vi "UiSchematic_gas.vi"() -> ()   [LabVIEW 2011]
uses:
  Pumpe.ctl
  Output - Cluster gas.ctl
panel:
  out "B2G1 HR V1":bool
  out "Fab2 MR V1":bool
  out "B2G1 MR V1":bool
  out "B2G2 T2 V1":bool
  out "B2G2 MR V1":bool
  out "B2G1 T2 V1":bool
  out "Fab1 BL V1":bool
  out "Fab1 HR V1":bool
  out "Fab1 MR V1":bool
  out "Fab2 HR V1":bool
  out "DS-2 [bar]":dbl format="%.4g"
  out "GZ-1 [l]":dbl format="%.2f"
  out "DS-1 [bar]":dbl format="%.4g"
  out "TS-1 [°C]":dbl format="%.2g"
  out "cRio":timestamp
  out "GM P-2":bool
  out "PC":timestamp
  in  "stop cRIO":bool
  out "GM V-1":bool
  out "GM V-4":bool
  out "GM V-3":bool
  out "GM V-2":bool
  out "GA1":timestamp caption="GA-1"
  out "h2 [%]":dbl format="%.2g"
  out "co2 [%]":dbl format="%.2g"
  out "ch4 [%]":dbl format="%.2g"
  out "GM P-1":T1
  out "B2G1 HR V1.1":bool
  out "Fab2 MR V1.1":bool
  out "B2G1 MR V1.1":bool
  out "B2G2 T2 V1.1":bool
  out "B2G2 MR V1.1":bool
  out "B2G1 T2 V1.1":bool
  out "Fab1 BL V1.1":bool
  out "Fab1 HR V1.1":bool
  out "Fab1 MR V1.1":bool
  out "Fab2 HR V1.1":bool
  in  "Output Var gas":refnum<k21>="ni.var.psp://10.27.40.21/variables - gas/data - network - gas"
  in  "stop":bool
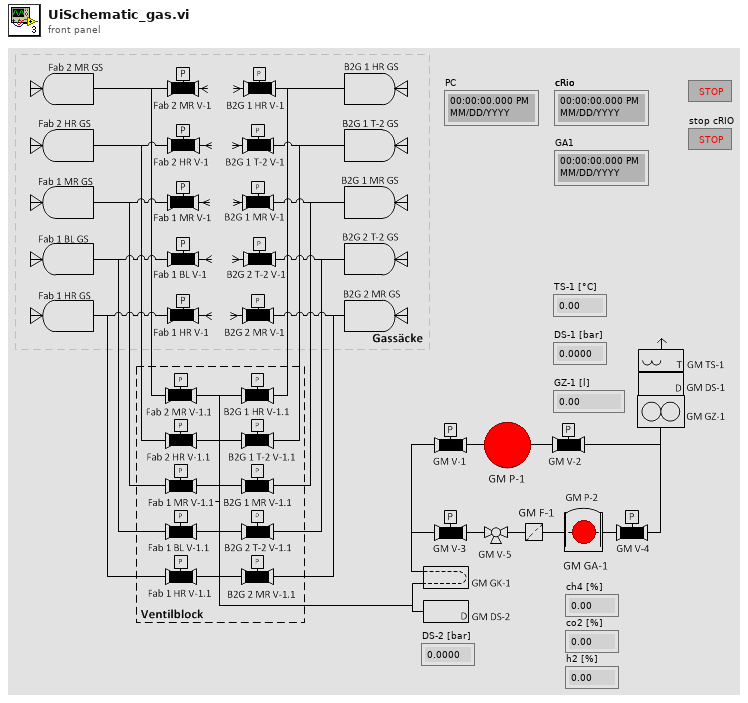
[diagram p1: front panel]
types:
  T1 = typedef "Pumpe.ctl" = bool
  T2 = typedef "Output - Cluster gas.ctl" = cluster{"B2G2 MR V1.1 AUF":bool, "B2G2 MR V1.1 ZU":bool, "B2G2 MR V1 AUF":bool, "B2G2 MR V1 ZU":bool, "B2G1 T2 V1 AUF":bool, "B2G1 T2 V1 ZU":bool, "B2G1 T2 V1.1 AUF":bool, "B2G1 T2 V1.1 ZU":bool, "B2G2 T2 V1 AUF":bool, "B2G2 T2 V1 ZU":bool, "B2G2 T2 V1.1 ZU":bool, "B2G2 T2 V1.1 AUF":bool, "B2G1 MR V1 AUF":bool, "B2G1 MR V1 ZU":bool, "B2G1 MR V1.1 AUF":bool, "B2G1 MR V1.1 ZU":bool, "B2G1 HR V1 AUF":bool, "B2G1 HR V1 ZU":bool, "B2G1 HR V1.1 AUF":bool, "B2G1 HR V1.1 ZU":bool, "Fab1 HR V1 AUF":bool, "Fab1 HR V1 ZU":bool, "Fab1 HR V1.1 AUF":bool, "Fab1 HR V1.1 ZU":bool, "Fab1 MR V1 AUF":bool, "Fab1 MR V1 ZU":bool, "Fab1 MR V1.1 AUF":bool, "Fab1 MR V1.1 ZU":bool, "Fab1 BL V1 AUF":bool, "Fab1 BL V1 ZU":bool, "Fab1 BL V1.1 AUF":bool, "Fab1 BL V1.1 ZU":bool, "Fab2 HR V1 AUF":bool, "Fab2 HR V1 ZU":bool, "Fab2 HR V1.1 AUF":bool, "Fab2 HR V1.1 ZU":bool, "Fab2 MR V1 AUF":bool, "Fab2 MR V1 ZU":bool, "Fab2 MR V1.1 AUF":bool, "Fab2 MR V1.1 ZU":bool, "GA1 ch4":dbl, "GA1 co2":dbl, "GA1 h2":dbl, "GM P1 RUN":bool, "GA1 timestamp":timestamp, "GM V-1 AUF":bool, "GM V-1 ZU":bool, "GM V-2 AUF":bool, "GM V-2 ZU":bool, "GM V-3 AUF":bool, "GM V-3 ZU":bool, "GM V-4 AUF":bool, "GM V-4 ZU":bool, "GM P2 RUN":bool, "GM GZ-1 [l]":dbl, "GM DS-2 [bar]":dbl, "GM DS-1 [bar]":dbl, "GM TS-1 [°C]":dbl}
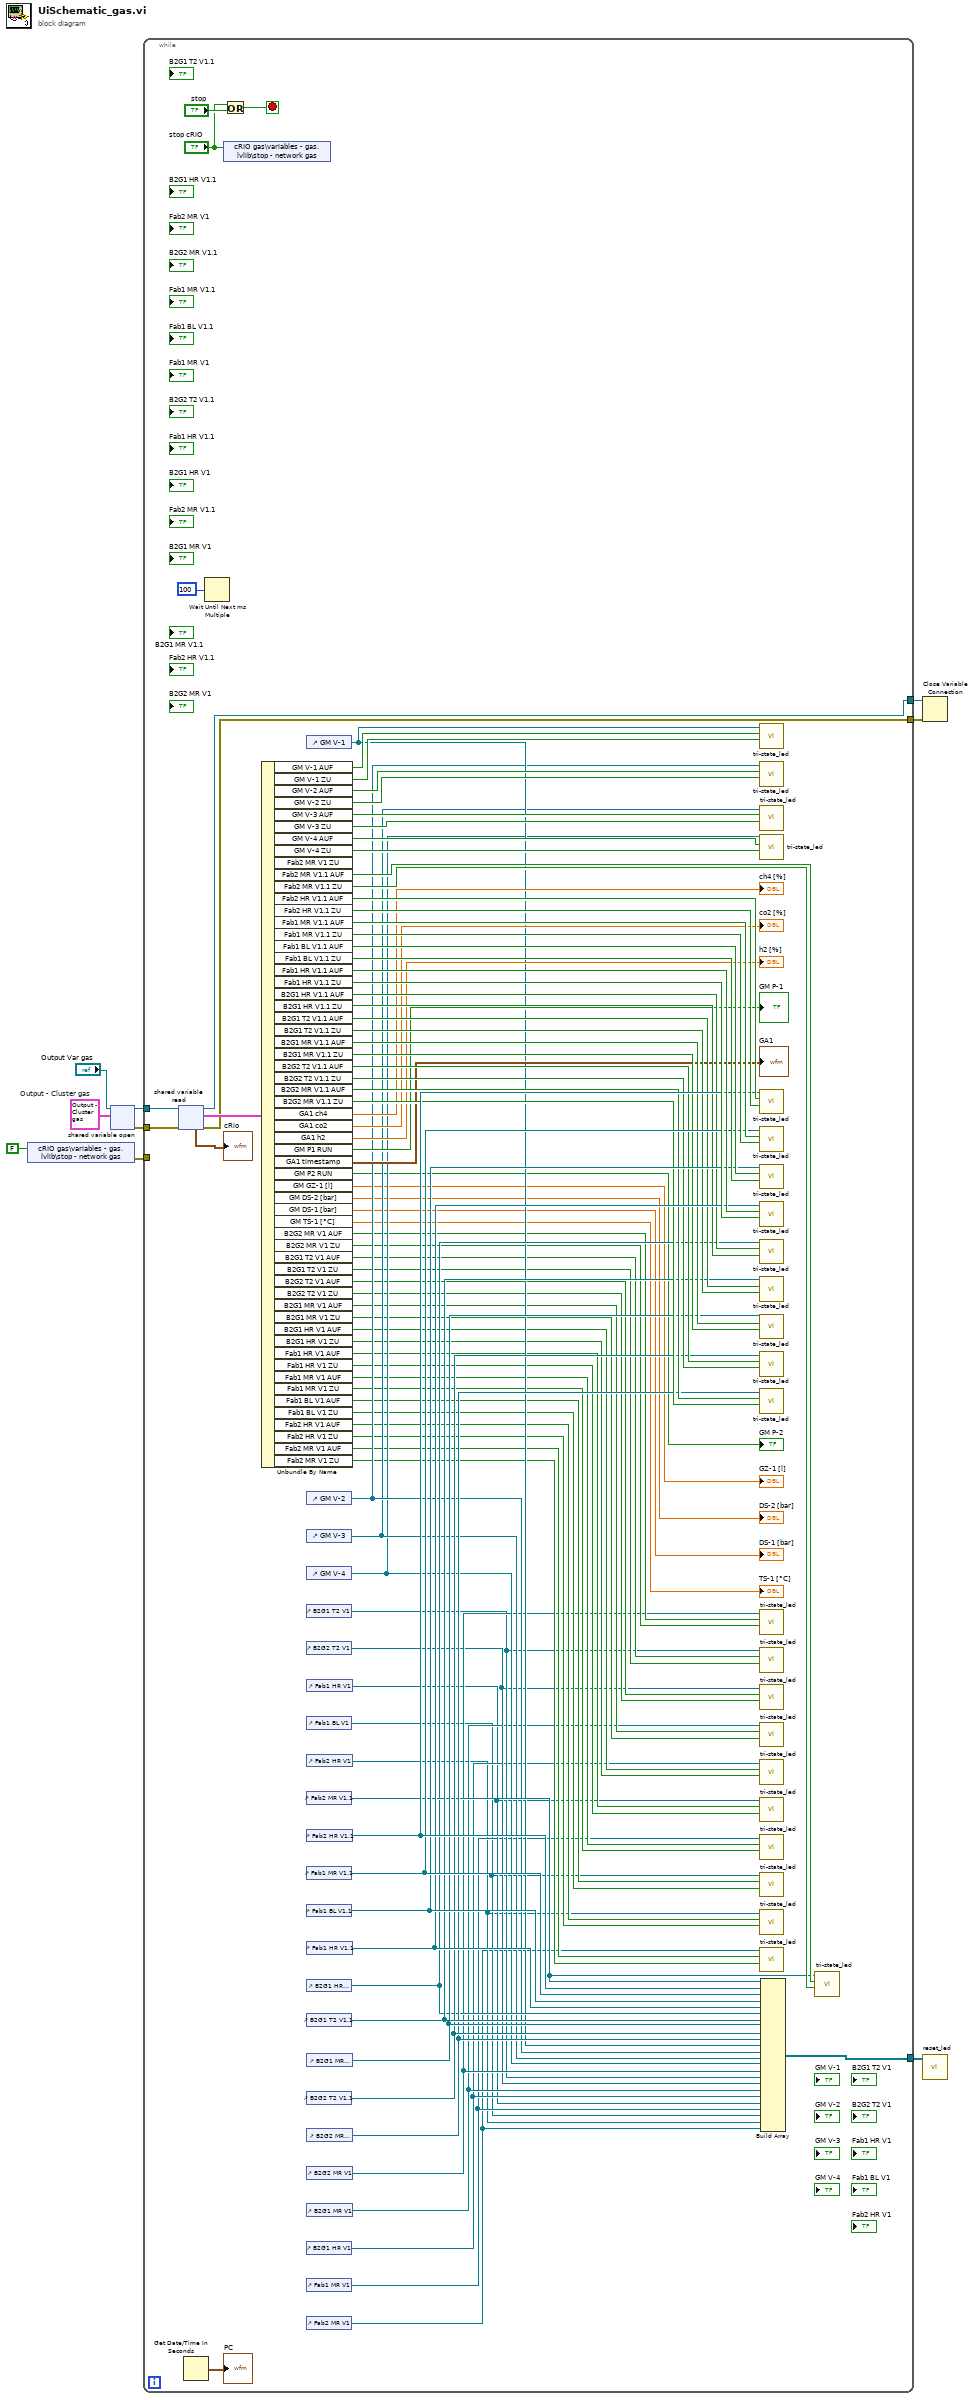
[diagram p0: block diagram]
diagram:
  w6 = T2 {"B2G2 MR V1.1 AUF"=FALSE, "B2G2 MR V1.1 ZU"=FALSE, "B2G2 MR V1 AUF"=FALSE, "B2G2 MR V1 ZU"=FALSE, "B2G1 T2 V1 AUF"=FALSE, "B2G1 T2 V1 ZU"=FALSE, "B2G1 T2 V1.1 AUF"=FALSE, "B2G1 T2 V1.1 ZU"=FALSE, "B2G2 T2 V1 AUF"=FALSE, "B2G2 T2 V1 ZU"=FALSE, "B2G2 T2 V1.1 ZU"=FALSE, "B2G2 T2 V1.1 AUF"=FALSE, "B2G1 MR V1 AUF"=FALSE, "B2G1 MR V1 ZU"=FALSE, "B2G1 MR V1.1 AUF"=FALSE, "B2G1 MR V1.1 ZU"=FALSE, "B2G1 HR V1 AUF"=FALSE, "B2G1 HR V1 ZU"=FALSE, "B2G1 HR V1.1 AUF"=FALSE, "B2G1 HR V1.1 ZU"=FALSE, "Fab1 HR V1 AUF"=FALSE, "Fab1 HR V1 ZU"=FALSE, "Fab1 HR V1.1 AUF"=FALSE, "Fab1 HR V1.1 ZU"=FALSE, "Fab1 MR V1 AUF"=FALSE, "Fab1 MR V1 ZU"=FALSE, "Fab1 MR V1.1 AUF"=FALSE, "Fab1 MR V1.1 ZU"=FALSE, "Fab1 BL V1 AUF"=FALSE, "Fab1 BL V1 ZU"=FALSE, "Fab1 BL V1.1 AUF"=FALSE, "Fab1 BL V1.1 ZU"=FALSE, "Fab2 HR V1 AUF"=FALSE, "Fab2 HR V1 ZU"=FALSE, "Fab2 HR V1.1 AUF"=FALSE, "Fab2 HR V1.1 ZU"=FALSE, "Fab2 MR V1 AUF"=FALSE, "Fab2 MR V1 ZU"=FALSE, "Fab2 MR V1.1 AUF"=FALSE, "Fab2 MR V1.1 ZU"=FALSE, "GA1 ch4"=0.0, "GA1 co2"=0.0, "GA1 h2"=0.0, "GM P1 RUN"=FALSE, "GA1 timestamp"=timestamp(0 s since 1904-01-01), "GM V-1 AUF"=FALSE, "GM V-1 ZU"=FALSE, "GM V-2 AUF"=FALSE, "GM V-2 ZU"=FALSE, "GM V-3 AUF"=FALSE, "GM V-3 ZU"=FALSE, "GM V-4 AUF"=FALSE, "GM V-4 ZU"=FALSE, "GM P2 RUN"=FALSE, "GM GZ-1 [l]"=0.0, "GM DS-2 [bar]"=0.0, "GM DS-1 [bar]"=0.0, "GM TS-1 [°C]"=0.0}  # Output - Cluster gas
  n1 = shared-variable "cRIO gas\\variables - gas.lvlib\\stop - network gas"(FALSE ("stop - network gas")) -> (error out=w2:errorcluster)  [unwired: 1 in]
  n2 = shared-variable-open("Output Var gas", w6) -> (w4:refnum<k21>, w3:errorcluster)  [unwired: 2 in]
  n3 = while {
    tunnel: w4 -> [w103]
    tunnel: [w102] -> w8
    tunnel: w3 -> [w100]
    tunnel: [w99] -> w7
    tunnel: [w83] -> w5
    tunnel: w2 -> [_]
    stop <- w49 stop-if-true
    n4 = shared-variable-read(w103, w100) -> (w102:refnum<k21>, w99:errorcluster, w101:T2, →"cRio":timestamp)
    n5 = Get Date/Time In Seconds() -> (seconds since 1Jan1904=→"PC":timestamp)
    n6 = Wait Until Next ms Multiple(millisecond multiple=u32 100) -> ()  [unwired: 1 out]
    n7 = Or(x="stop cRIO", y="stop") -> (x .or. y?=w49:bool)
    n8 = shared-variable "cRIO gas\\variables - gas.lvlib\\stop - network gas"("stop cRIO") -> ()  [unwired: 1 in, 1 out]
    n9 = Unbundle By Name(w101) -> ("GM V-1 AUF"=w61:bool, "GM V-1 ZU"=w60:bool, "GM V-2 AUF"=w59:bool, "GM V-2 ZU"=w58:bool, "GM V-3 AUF"=w57:bool, "GM V-3 ZU"=w56:bool, "GM V-4 AUF"=w55:bool, "GM V-4 ZU"=w54:bool, "Fab2 MR V1.1 AUF"=w97:bool, "Fab2 MR V1.1 ZU"=w96:bool, "Fab2 HR V1.1 AUF"=w95:bool, "Fab2 HR V1.1 ZU"=w94:bool, "Fab1 MR V1.1 AUF"=w93:bool, "Fab1 MR V1.1 ZU"=w92:bool, "Fab1 BL V1.1 AUF"=w91:bool, "Fab1 BL V1.1 ZU"=w90:bool, "Fab1 HR V1.1 AUF"=w89:bool, "Fab1 HR V1.1 ZU"=w88:bool, "B2G1 HR V1.1 AUF"=w82:bool, "B2G1 HR V1.1 ZU"=w81:bool, "B2G1 T2 V1.1 AUF"=w80:bool, "B2G1 T2 V1.1 ZU"=w79:bool, "B2G1 MR V1.1 AUF"=w78:bool, "B2G1 MR V1.1 ZU"=w77:bool, "B2G2 T2 V1.1 AUF"=w76:bool, "B2G2 T2 V1.1 ZU"=w75:bool, "B2G2 MR V1.1 AUF"=w74:bool, "B2G2 MR V1.1 ZU"=w73:bool, "GA1 ch4"=→"ch4 [%]":dbl, "GA1 co2"=→"co2 [%]":dbl, "GA1 h2"=→"h2 [%]":dbl, "GM P1 RUN"=→"GM P-1":bool, "GA1 timestamp"=→"GA1":timestamp, "GM P2 RUN"=→"GM P-2":bool, "GM GZ-1 [l]"=→"GZ-1 [l]":dbl, "GM DS-2 [bar]"=→"DS-2 [bar]":dbl, "GM DS-1 [bar]"=→"DS-1 [bar]":dbl, "GM TS-1 [°C]"=→"TS-1 [°C]":dbl, "B2G2 MR V1 AUF"=w39:bool, "B2G2 MR V1 ZU"=w38:bool, "B2G1 T2 V1 AUF"=w37:bool, "B2G1 T2 V1 ZU"=w36:bool, "B2G2 T2 V1 AUF"=w35:bool, "B2G2 T2 V1 ZU"=w34:bool, "B2G1 MR V1 AUF"=w33:bool, "B2G1 MR V1 ZU"=w32:bool, "B2G1 HR V1 AUF"=w31:bool, "B2G1 HR V1 ZU"=w30:bool, "Fab1 HR V1 AUF"=w29:bool, "Fab1 HR V1 ZU"=w28:bool, "Fab1 MR V1 AUF"=w27:bool, "Fab1 MR V1 ZU"=w26:bool, "Fab1 BL V1 AUF"=w25:bool, "Fab1 BL V1 ZU"=w24:bool, "Fab2 HR V1 AUF"=w23:bool, "Fab2 HR V1 ZU"=w22:bool, "Fab2 MR V1 AUF"=w21:bool, "Fab2 MR V1 ZU"=w20:bool)  [unwired: 1 out]
    n10 = control-ref of="GM V-1"() -> (w53:refnum<vi>)
    n11 = control-ref of="GM V-2"() -> (w52:refnum<vi>)
    n12 = control-ref of="GM V-3"() -> (w51:refnum<vi>)
    n13 = control-ref of="GM V-4"() -> (w50:refnum<vi>)
    n14 = control-ref of="B2G1 T2 V1"() -> (w18:refnum<vi>)
    n15 = control-ref of="B2G2 T2 V1"() -> (w17:refnum<vi>)
    n16 = control-ref of="Fab1 BL V1"() -> (w12:refnum<vi>)
    n17 = control-ref of="Fab2 MR V1.1"() -> (w68:refnum<vi>)
    n18 = control-ref of="Fab1 MR V1.1"() -> (w86:refnum<vi>)
    n19 = control-ref of="Fab1 BL V1.1"() -> (w85:refnum<vi>)
    n20 = control-ref of="B2G1 HR V1.1"() -> (w67:refnum<vi>)
    n21 = control-ref of="B2G1 T2 V1.1"() -> (w72:refnum<vi>)
    n22 = control-ref of="B2G2 T2 V1.1"() -> (w70:refnum<vi>)
    n23 = control-ref of="B2G1 HR V1"() -> (w15:refnum<vi>)
    n24 = control-ref of="Fab1 MR V1"() -> (w13:refnum<vi>)
    n25 = control-ref of="Fab2 MR V1"() -> (w10:refnum<vi>)
    n26 = control-ref of="Fab1 HR V1"() -> (w14:refnum<vi>)
    n27 = control-ref of="Fab2 HR V1"() -> (w11:refnum<vi>)
    n28 = control-ref of="Fab2 HR V1.1"() -> (w87:refnum<vi>)
    n29 = control-ref of="Fab1 HR V1.1"() -> (w84:refnum<vi>)
    n30 = control-ref of="B2G1 MR V1.1"() -> (w71:refnum<vi>)
    n31 = control-ref of="B2G2 MR V1.1"() -> (w69:refnum<vi>)
    n32 = control-ref of="B2G2 MR V1"() -> (w19:refnum<vi>)
    n33 = control-ref of="B2G1 MR V1"() -> (w16:refnum<vi>)
    n34 = call "tri-state_led.vi"("CLOSE"=w60, "OPEN"=w61, "ref in"=w53) -> ()  [unwired: 9 in]
    n35 = call "tri-state_led.vi"("CLOSE"=w58, "OPEN"=w59, "ref in"=w52) -> ()  [unwired: 9 in]
    n36 = call "tri-state_led.vi"("CLOSE"=w56, "OPEN"=w57, "ref in"=w51) -> ()  [unwired: 9 in]
    n37 = call "tri-state_led.vi"("CLOSE"=w54, "OPEN"=w55, "ref in"=w50) -> ()  [unwired: 9 in]
    n38 = call "tri-state_led.vi"("CLOSE"=w94, "OPEN"=w95, "ref in"=w87) -> ()  [unwired: 9 in]
    n39 = call "tri-state_led.vi"("CLOSE"=w92, "OPEN"=w93, "ref in"=w86) -> ()  [unwired: 9 in]
    n40 = call "tri-state_led.vi"("CLOSE"=w90, "OPEN"=w91, "ref in"=w85) -> ()  [unwired: 9 in]
    n41 = call "tri-state_led.vi"("CLOSE"=w88, "OPEN"=w89, "ref in"=w84) -> ()  [unwired: 9 in]
    n42 = call "tri-state_led.vi"("CLOSE"=w81, "OPEN"=w82, "ref in"=w67) -> ()  [unwired: 9 in]
    n43 = call "tri-state_led.vi"("CLOSE"=w79, "OPEN"=w80, "ref in"=w72) -> ()  [unwired: 9 in]
    n44 = call "tri-state_led.vi"("CLOSE"=w77, "OPEN"=w78, "ref in"=w71) -> ()  [unwired: 9 in]
    n45 = call "tri-state_led.vi"("CLOSE"=w75, "OPEN"=w76, "ref in"=w70) -> ()  [unwired: 9 in]
    n46 = call "tri-state_led.vi"("CLOSE"=w73, "OPEN"=w74, "ref in"=w69) -> ()  [unwired: 9 in]
    n47 = call "tri-state_led.vi"("CLOSE"=w38, "OPEN"=w39, "ref in"=w19) -> ()  [unwired: 9 in]
    n48 = call "tri-state_led.vi"("CLOSE"=w36, "OPEN"=w37, "ref in"=w18) -> ()  [unwired: 9 in]
    n49 = call "tri-state_led.vi"("CLOSE"=w34, "OPEN"=w35, "ref in"=w17) -> ()  [unwired: 9 in]
    n50 = call "tri-state_led.vi"("CLOSE"=w32, "OPEN"=w33, "ref in"=w16) -> ()  [unwired: 9 in]
    n51 = call "tri-state_led.vi"("CLOSE"=w30, "OPEN"=w31, "ref in"=w15) -> ()  [unwired: 9 in]
    n52 = call "tri-state_led.vi"("CLOSE"=w28, "OPEN"=w29, "ref in"=w14) -> ()  [unwired: 9 in]
    n53 = call "tri-state_led.vi"("CLOSE"=w26, "OPEN"=w27, "ref in"=w13) -> ()  [unwired: 9 in]
    n54 = call "tri-state_led.vi"("CLOSE"=w24, "OPEN"=w25, "ref in"=w12) -> ()  [unwired: 9 in]
    n55 = call "tri-state_led.vi"("CLOSE"=w22, "OPEN"=w23, "ref in"=w11) -> ()  [unwired: 9 in]
    n56 = call "tri-state_led.vi"("CLOSE"=w20, "OPEN"=w21, "ref in"=w10) -> ()  [unwired: 9 in]
    n57 = Build Array(w68, w87, w86, w85, w84, w67, w72, w71, w70, w69, w53, w52, w51, w50, w19, w18, w17, w16, w15, w14, w13, w12, w11, w10) -> (w83:refnum<vi>[])
    n58 = call "tri-state_led.vi"("CLOSE"=w96, "OPEN"=w97, "ref in"=w68) -> ()  [unwired: 9 in]
  }
  n59 = Close Variable Connection(8:w7, 11:w8) -> ()  [unwired: 1 out]
  n60 = call "reset_led.vi"("Array"=w5) -> ()  [unwired: 11 in]
